vi "AIM Multichannel Tx and RX PARAM Constants.vi"(1 "Transfer Type":enum16{"Acyclic", "Scheduled"}(ring)) -> (0 "Parameters (3D Array)":i32[][][](array[numeric]))   [LabVIEW 2020]
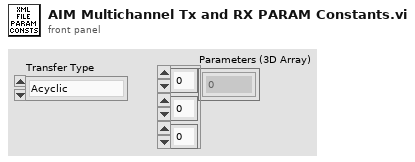
[diagram p1: front panel]
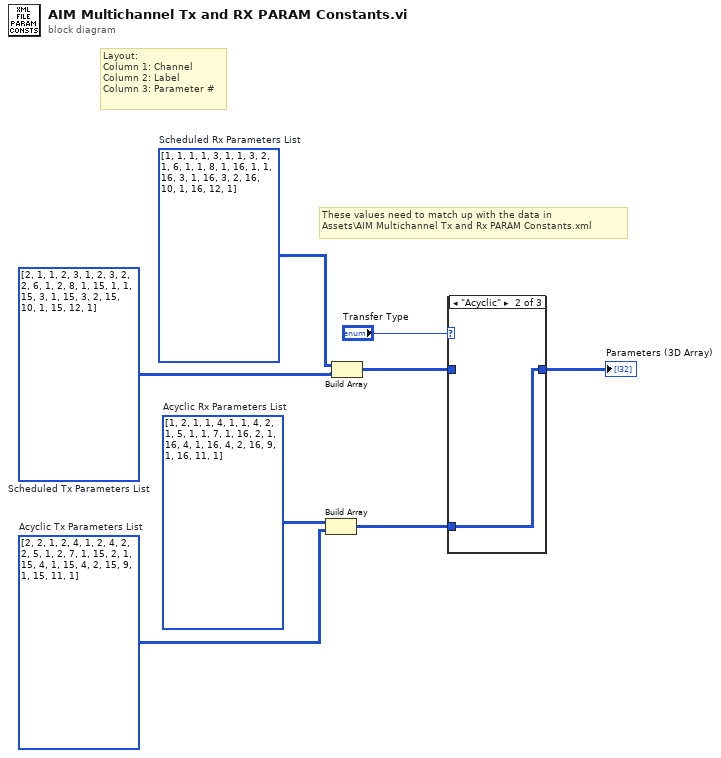
[diagram p0: block diagram]
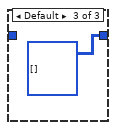
[diagram p3: hidden frame]
diagram:
  w2 = i32[][] [[1, 2, 1], [1, 4, 1], [1, 4, 2], [1, 5, 1], [1, 7, 1], [16, 2, 1], [16, 4, 1], [16, 4, 2], [16, 9, 1], [16, 11, 1]]  # Acyclic Rx Parameters List
  w4 = i32[][] [[1, 1, 1], [1, 3, 1], [1, 3, 2], [1, 6, 1], [1, 8, 1], [16, 1, 1], [16, 3, 1], [16, 3, 2], [16, 10, 1], [16, 12, 1]]  # Scheduled Rx Parameters List
  w1 = i32[][] [[2, 2, 1], [2, 4, 1], [2, 4, 2], [2, 5, 1], [2, 7, 1], [15, 2, 1], [15, 4, 1], [15, 4, 2], [15, 9, 1], [15, 11, 1]]  # Acyclic Tx Parameters List
  w3 = i32[][] [[2, 1, 1], [2, 3, 1], [2, 3, 2], [2, 6, 1], [2, 8, 1], [15, 1, 1], [15, 3, 1], [15, 3, 2], [15, 10, 1], [15, 12, 1]]  # Scheduled Tx Parameters List
  # "These values need to match up with the data in\nAssets\\AIM Multichannel Tx and Rx PARAM Constants.xml"
  # "Layout:\nColumn 1: Channel\nColumn 2: Label\nColumn 3: Parameter #"
  n1 = Build Array(w2, w1) -> (w5:i32[][][])
  n2 = Build Array(w4, w3) -> (w6:i32[][][])
  n3 = case shown="\"Acyclic\"" "Transfer Type" {
    tunnel: [w9 w10 i32[][][] [] ("Parameters (3D Array)")] -> w7
    tunnel: w6 -> [w9 _ _]
    tunnel: w5 -> [_ w10 _]
    frame "Scheduled" {
    }
    frame "Acyclic" {
    }
    frame Default {
    }
  }
  "Parameters (3D Array)" <- w7
